vi "ResetVIs.vi"() -> ()   [LabVIEW 2019]
panel:
  in  "Reset?":bool=TRUE
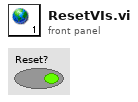
[diagram p1: front panel]
diagram:
